vi "APC_9049_PPhaseCorrection.vi"(0 "UsePcylDatabase":bool, 2 "AIdata [bar]":dbl[][](array[numeric])=array8x7200[57600 elements]) -> (1 "SystemP [bar]":dbl format="%0.2f", 3 "PrechamberPeakDiff [bar]":dbl format="%0.2f", 4 "ExhaustP [bar]":dbl format="%0.2f", 5 "RawPcyl [bar]":dbl[][](array[numeric]), 6 "PhaseCompPcyl [bar]":dbl[][](array[numeric]), 7 "PhaseCompPexh [bar]":dbl[][](array[numeric]))   [LabVIEW 2020]
doc: "This example demonstrates the procedure required to apply different NI-DAQmx Custom Scales to each virtual channel in a task. A DAQmx Task Property Node (Functions >> NI Measurements >> DAQmx - Data Acquisition >> DAQmx Advanced Task Options) is used to obtain the task's virtual channels. A DAQmx Channel Property Node (Functions >> NI Measurements >> DAQmx - Data Acquisition) is then used to set the custom scale for each virtual channel in the task.\n\nThe \"DAQmx Create Scale\" VI creates a custom scale for each channel in the channel list. *Note, make sure your Minimum and Maximum channel parameters are consistent with the range the scale will create."
uses:
  <vilib>/Analysis/baseanly.llb/Mean (DBL).vi
  <vilib>/Analysis/NI_AALBase.lvlib
panel:
  out "TDC fail":bool
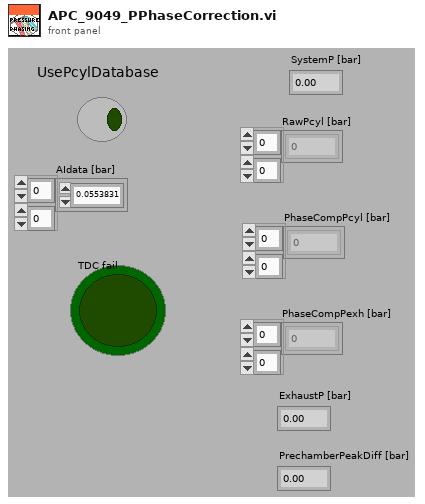
[diagram p1: front panel]
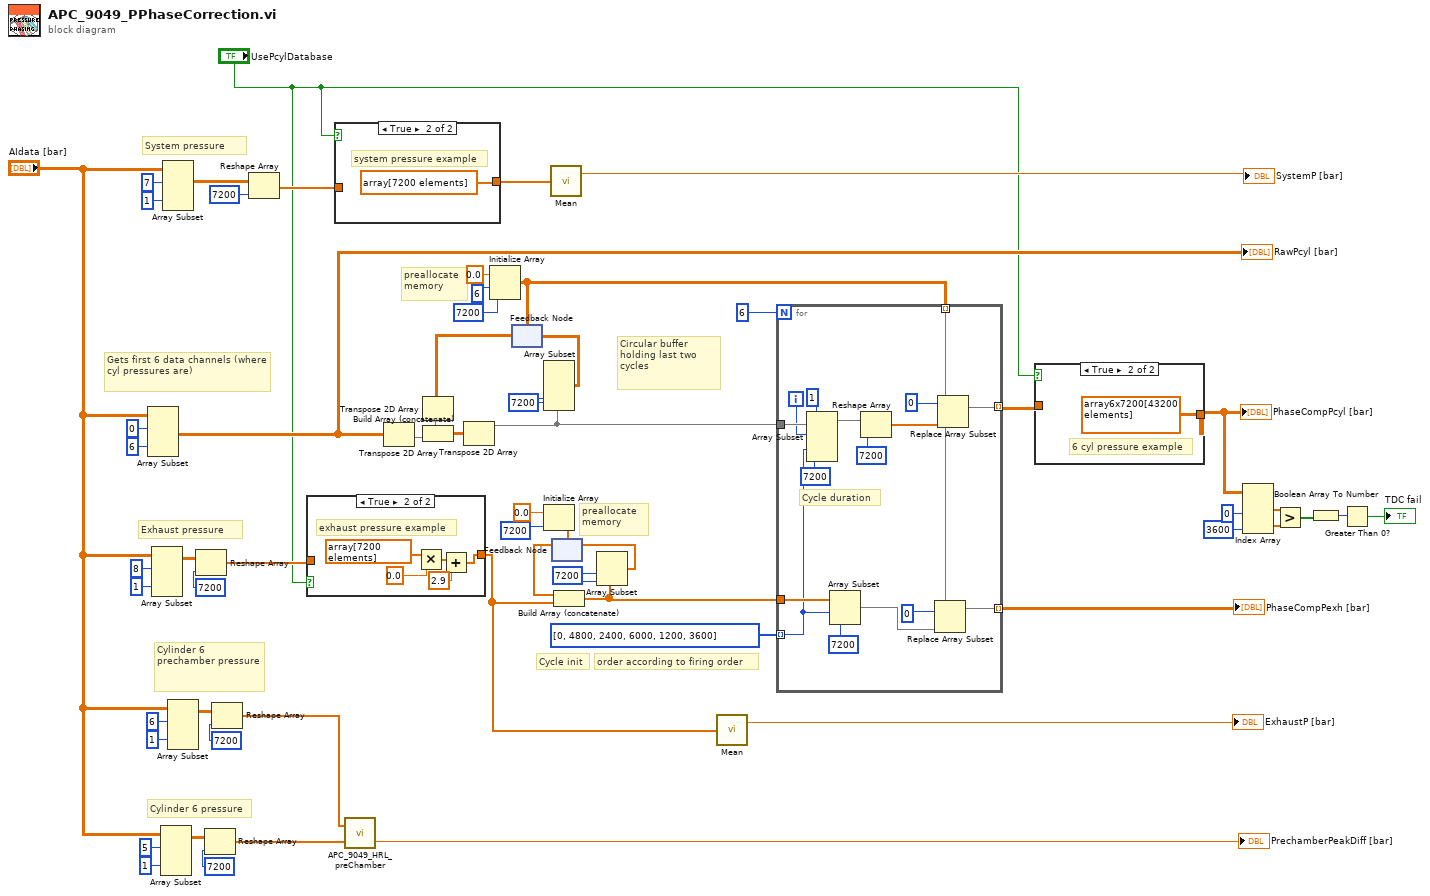
[diagram p0: block diagram]
diagram:
  w29 = 7200 ("index")
  w22 = 7200 ("length")
  # "Cylinder 6 prechamber pressure"
  # "Cylinder 6 pressure"
  # "Exhaust pressure"
  # "preallocate memory"
  # "System pressure"
  # "Gets first 6 data channels (where cyl pressures are)"
  # "order according to firing order"
  # "preallocate memory"
  # "Cycle init"
  # "Circular buffer holding last two cycles"
  n1 = Array Subset(array="AIdata [bar]", index (row)=0 ("index"), length (row)=6 ("length")) -> (w40:dbl[][])  [unwired: 2 in]
  "RawPcyl [bar]" <- w40
  n2 = Array Subset(array="AIdata [bar]", index (row)=8 ("index"), index (col)=1 ("length")) -> (w30:dbl[][])  [unwired: 2 in]
  n3 = Array Subset(array="AIdata [bar]", index (row)=5 ("index"), index (col)=1 ("length")) -> (w9:dbl[][])  [unwired: 2 in]
  n4 = Array Subset(array="AIdata [bar]", index (row)=7 ("index"), length (row)=1 ("length")) -> (w52:dbl[][])  [unwired: 2 in]
  n5 = Array Subset(array="AIdata [bar]", index (row)=6 ("index"), index (col)=1 ("length")) -> (w4:dbl[][])  [unwired: 2 in]
  n6 = Reshape Array(w30, 7200 ("dimension size")) -> (w27:dbl[])
  n7 = Reshape Array(w9, 7200 ("dimension size")) -> (w8:dbl[])
  n8 = Reshape Array(w4, 7200 ("dimension size")) -> (w2:dbl[])
  n9 = Reshape Array(w52, 7200 ("dimension size")) -> (w24:dbl[])
  n10 = case shown="True" "UsePcylDatabase" {
    tunnel: w27 -> [w61 _]
    tunnel: [w61 w64] -> w25
    frame False {
    }
    frame True {
      # "exhaust pressure example"
      n11 = Multiply(x=dbl[] array[7200 elements] ("exhaust pressure"), y=0.0) -> (x*y=w65:dbl[])
      n12 = Add(x=w65, y=2.9) -> (x+y=w64:dbl[])
    }
  }
  n13 = case shown="True" "UsePcylDatabase" {
    tunnel: w24 -> [w67 _]
    tunnel: [w67 dbl[] array[7200 elements] ("exhaust pressure")] -> w23
    frame False {
    }
    frame True {
      # "system pressure example"
    }
  }
  n14 = call "APC_9049_HRL_preChamber.vi"("InCylPressure"=w8, "PrechamberPressure"=w2) -> ("peakPrechamberPdiff"=→"PrechamberPeakDiff [bar]":dbl)  [unwired: 1 out]
  n15 = Transpose 2D Array(2D array=w40) -> (transposed array=w47:dbl[][])
  n16 = Initialize Array(0.0 ("element"), 6 ("dimension size"), 7200 ("dimension size")) -> (w41:dbl[][])
  n17 = feedback #1(w41) -> (w43:dbl[][])
  n18 = Transpose 2D Array(2D array=w43) -> (transposed array=w46:dbl[][])
  n19 = Build Array (concatenate)(w46, w47) -> (w45:dbl[][])
  n20 = Transpose 2D Array(2D array=w45) -> (transposed array=w42:dbl[][])
  n21 = Array Subset(array=w42, index (col)=w22, length (col)=w22) -> (w44:dbl[][])  [unwired: 2 in]
  n22 = feedback-in #1(w44) -> ()
  n23 = Initialize Array(0.0 ("element"), 7200 ("dimension size")) -> (w33:dbl[])
  n24 = call-poly <vilib>:"Mean.vi"("X"=w23) -> ("mean"=→"SystemP [bar]":dbl)  [unwired: 1 out]
  n25 = feedback #2(w33) -> (w36:dbl[])
  n26 = Build Array (concatenate)(w36, w25) -> (w38:dbl[])
  n27 = Array Subset(array=w38, index=w29, length=w29) -> (w37:dbl[])
  n28 = feedback-in #2(w37) -> ()
  n29 = call-poly <vilib>:"Mean.vi"("X"=w25) -> ("mean"=→"ExhaustP [bar]":dbl)  [unwired: 1 out]
  n30 = for {
    N: 6 -> [_]
    tunnel: w42 -> [w84]
    tunnel: i32[] [0, 4800, 2400, 6000, 1200, 3600] ("index") -> [w73] mode=indexing
    tunnel: w41 -> [w70] mode=indexing
    tunnel: [w77] -> w28 mode=indexing
    tunnel: w38 -> [w75]
    tunnel: [w69] -> w26 mode=indexing
    i -> [w79]
    # "Cycle duration"
    n31 = Array Subset(array=w84, index (row)=w79, length (row)=1 ("length"), index (col)=w73, length (col)=7200 ("index")) -> (w83:dbl[][])
    n32 = Array Subset(array=w75, index=w73, length=7200) -> (w72:dbl[])
    n33 = Reshape Array(w83, 7200 ("dimension size")) -> (w82:dbl[])
    n34 = Replace Array Subset(array=w70, new element=w72, index=0) -> (w69:dbl[])
    n35 = Replace Array Subset(array=w70, new element=w82, index=0) -> (w77:dbl[])
  }
  "PhaseCompPexh [bar]" <- w26
  n36 = case shown="True" "UsePcylDatabase" {
    tunnel: [w85 dbl[][] array6x7200[43200 elements] ("6 P cyl example")] -> w20
    tunnel: w28 -> [w85 _]
    frame False {
    }
    frame True {
      # "6 cyl pressure example"
    }
  }
  "PhaseCompPcyl [bar]" <- w20
  n37 = Index Array(array=w20, index (col) #1=0 ("disabled index (col)"), index (col) #2=3600 ("index (col)")) -> (element #1=w17:dbl[], element #2=w16:dbl[])  [unwired: 2 in]
  n38 = Greater?(x=w17, y=w16) -> (0:w15:bool[])
  n39 = Boolean Array To Number(Boolean array=w15) -> (number=w14:u32)
  n40 = Greater Than 0?(x=w14) -> (x > 0?=→"TDC fail":bool)
